vi "ResetChainValues.vi"(8 "error in (no error)":errorcluster, 10 "Chains":u8[](array[numeric]), 11 "ControlState in":T1 {"ChainMask" format="0x%02x"}) -> (0 "error out":errorcluster, 2 "ChainMask":u8 format="0x%02x", 3 "ControlState out":T1 {"ChainMask" format="0x%02x"})   [LabVIEW 2018, in "ArduinoSerialBling.lvlib"]
uses:
  ArduinoSerialBling.lvlib
  ControlState.ctl
  ConnectionType.ctl
  UdpConnection.ctl
  ChainState.ctl
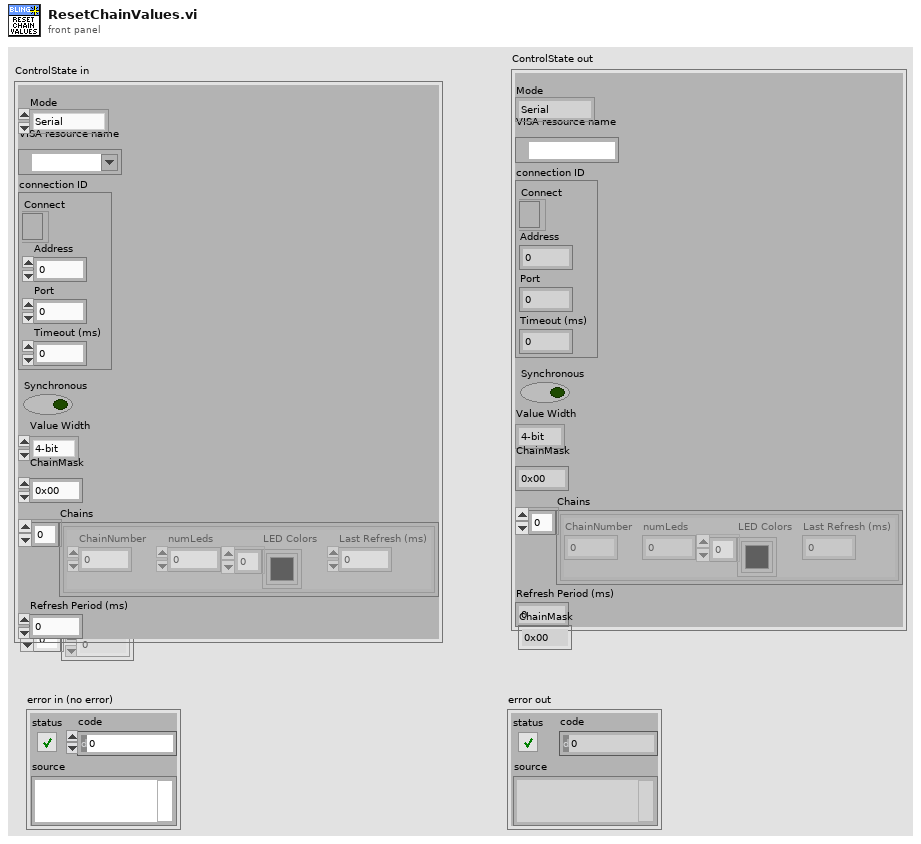
[diagram p1: front panel]
types:
  T1 = typedef "ArduinoSerialBling.lvlib/ControlState.ctl" = cluster{"Mode":T2, "VISA resource name":refnum<visa-resource-name>, "connection ID":T3, "Synchronous":bool, "Value Width":enum16{"4-bit", "8-bit"}, "ChainMask":u8, "Chains":T4[], "Refresh Period (ms)":u32}
  T2 = typedef "ConnectionType.ctl" = enum16{"Serial", "Ethernet", "Offline"}
  T3 = typedef "UdpConnection.ctl" = cluster{"Connect":refnum<k16>, "Address":u32, "Port":u16, "Timeout (ms)":i32}
  T4 = typedef "ArduinoSerialBling.lvlib/ChainState.ctl" = cluster{"ChainNumber":u8, "numLeds":u8, "LED Colors":u32[], "Last Refresh (ms)":u32}
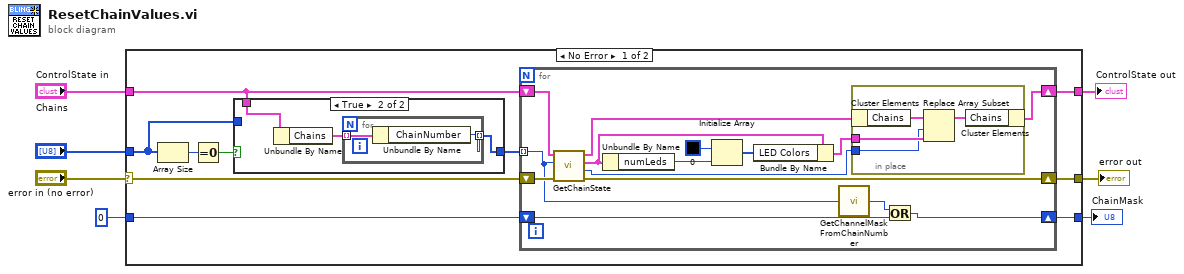
[diagram p0: block diagram]
diagram:
  n1 = case shown="No Error" "error in (no error)" {
    selector: "error in (no error)" -> [w13 w44]
    tunnel: "Chains" -> [w10 _]
    tunnel: "ControlState in" -> [w8 w45]
    tunnel: [w17 w44] -> w5
    tunnel: [w16 w45] -> w4
    tunnel: u8 0 -> [w15 w43]
    tunnel: [w14 w43] -> w2
    frame No Error {
      n2 = Array Size(array=w10) -> (size(s)=w12:i32)
      n3 = Equal To 0?(x=w12) -> (x = 0?=w11:bool)
      n4 = case shown="True" w11 {
        tunnel: w10 -> [w18 _]
        tunnel: [w18 w19] -> w9
        tunnel: w8 -> [_ w21]
        frame False {
        }
        frame True {
          n5 = Unbundle By Name(w21) -> ("Chains"=w20:T4[])
          n6 = for {
            tunnel: w20 -> [w23] mode=indexing
            tunnel: [w22] -> w19 mode=indexing
            n7 = Unbundle By Name(w23) -> ("ChainNumber"=w22:u8)
          }
        }
      }
      n8 = for {
        tunnel: w9 -> [w27] mode=indexing
        shift-right: [w28] -> w16
        shift-left: w8 -> [w37]
        shift-right: [w29] -> w17
        shift-left: w13 -> [w36]
        shift-right: [w24] -> w14
        shift-left: w15 -> [w25]
        n9 = call "GetChainState.vi"("error in (no error)"=w36, "ChainNumber"=w27, "ControlState in"=w37) -> ("error out"=w29:errorcluster, "ChainIndex"=w30:i32, "ChainState"=w34:T4, "ControlState out"=w32:T1)  [unwired: 5 in]
        n10 = Unbundle By Name(w34) -> ("numLeds"=w33:u8)
        n11 = Initialize Array(u32 0, w33) -> (w35:u32[])
        n12 = Bundle By Name(cluster=w34, "LED Colors"=w35) -> (w31:T4)
        n13 = call "GetChannelMaskFromChainNumber.vi"("ChainNumber"=w27) -> ("ChainMask"=w26:u8)
        n14 = in-place {
          in-place-border: w31 -> [w40]
          in-place-border: w30 -> [w39]
          n15 = in-place-cluster #1(w32) -> ("Chains"=w42:T4[])
          n16 = Replace Array Subset(array=w42, new element=w40, index=w39) -> (w41:T4[])
          n17 = in-place-cluster #1("Chains"=w41) -> (w28:T1)
        }
        n18 = Or(x=w26, y=w25) -> (x .or. y?=w24:u8)
      }
    }
    frame Error {
    }
  }
  "error out" <- w5
  "ControlState out" <- w4
  "ChainMask" <- w2
